vi "Point.vi"() -> ()   [LabVIEW 2011]
uses:
  <vilib>/Utility/miscctls.llb/LVPoint32TypeDef.ctl
  <vilib>/Utility/miscctls.llb/LVPositionTypeDef.ctl
panel:
  out "Content Rect Position":T1
  out "Position":T1
  out "Row":i32
  out "In Symbol?":bool
  out "In Bounds?":bool
  out "Coords":T2
  in  "stop":bool
  in  "Listbox":i32(listbox)
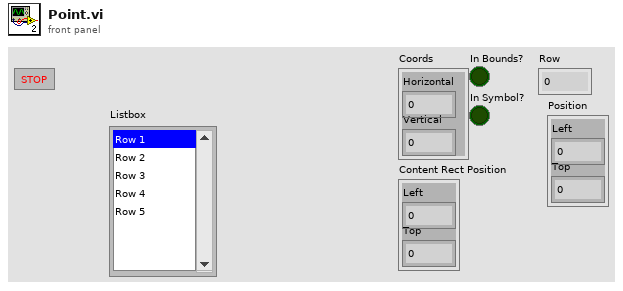
[diagram p1: front panel]
types:
  T1 = typedef "LVPositionTypeDef.ctl" = cluster{"Left":i32, "Top":i32}
  T2 = typedef "LVPoint32TypeDef.ctl" = cluster{"Horizontal":i32, "Vertical":i32}
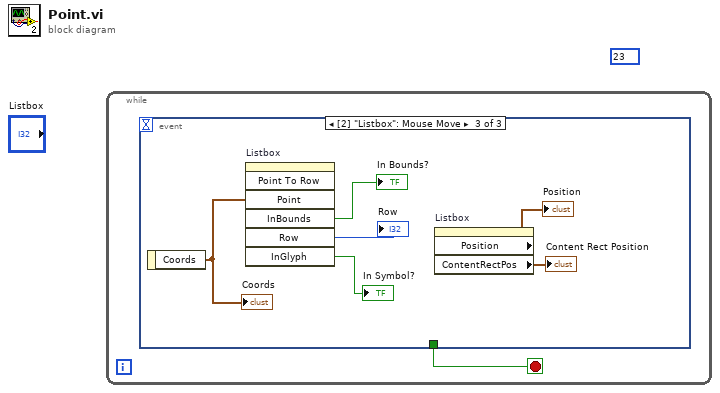
[diagram p0: block diagram]
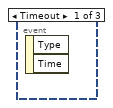
[diagram p2: hidden frame]
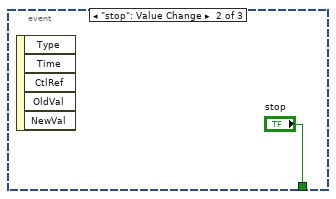
[diagram p3: hidden frame]
diagram:
  (unwired) 23
  n1 = while {
    stop <- w1 stop-if-true
    n2 = event shown="[2] \"Listbox\": Mouse Move" {
      selector: _ -> [_ _ _]
      dyn-events: _ -> [_ _ _]
      timeout: _ -> [_ _ _]
      tunnel: [_ "stop" _] -> w1
      event Timeout {
        n3 = event-data() -> ()  [unwired: 1 in, 2 out]
      }
      event "stop": Value Change {
        n4 = event-data() -> ()  [unwired: 1 in, 5 out]
      }
      event "Listbox": Mouse Move {
        n5 = event-data() -> ("Coords"=w8:T2)  [unwired: 1 in]
        "Coords" <- w8
        n6 = invoke on="Listbox" class="LstBox (strict)" method="Point To Row"("Point"=w8) -> ("InBounds"=→"In Bounds?":bool, "Row"=→"Row":i32, "InGlyph"=→"In Symbol?":bool)  [unwired: 6 in, 4 out]
        n7 = property on="Listbox" class="LstBox (strict)"() -> ("Position"=→"Position":T1, "ContentRectPos"=→"Content Rect Position":T1)  [unwired: 2 in, 2 out]
      }
    }
  }
